vi "Write Function Name.vi"(10 "Function Name":string, 11 "Find Devices of Specified Type Msg in":refnum<class "Find Devices of Specified Type Msg.lvclass">) -> (3 "Find Devices of Specified Type Msg out":refnum<class "Find Devices of Specified Type Msg.lvclass">)   [LabVIEW 2016, in "Controller Actor.lvlib" / "Find Devices of Specified Type Msg.lvclass"]
uses:
  <userlib>/Common Components/Controller/Messages/Find Devices of Specified Type Msg/Find Devices of Specified Type Msg.lvclass
  <userlib>/Common Components/Controller/Messages/Find Devices of Specified Type Msg/Find Devices of Specified Type Msg.lvclass/Find Devices of Specified Type Msg.ctl
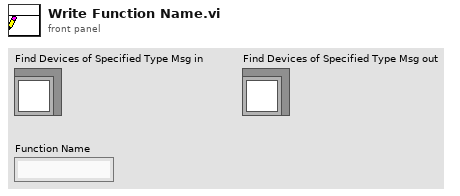
[diagram p1: front panel]
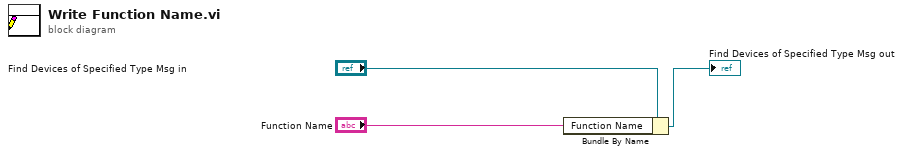
[diagram p0: block diagram]
diagram:
  n1 = Bundle By Name(cluster="Find Devices of Specified Type Msg in", "Function Name"="Function Name") -> (→"Find Devices of Specified Type Msg out":refnum<class "Find Devices of Specified Type Msg.lvclass">)
